vi "SLL DE DO LV2 Global.vi"(6 "DO State Array":bool[](array[boolean]), 7 "DO Option":T2, 8 "Error In":errorcluster, 9 "DO State":bool, 10 "DO Channel Name Array":T1[](array[typedef]), 11 "DO Channel Name":T1) -> (0 "error out":errorcluster, 2 "Digital Array Status":bool[](array[boolean]), 3 "Digital Line Status":bool, 4 "Element Wrote":string)   [LabVIEW 2013]
uses:
  Controls/SLL DE DO Global Options.ctl
  Controls/SLL DE List of Digital Outputs.ctl
  Controls/SLL DE DO Command LV2Global Options.ctl
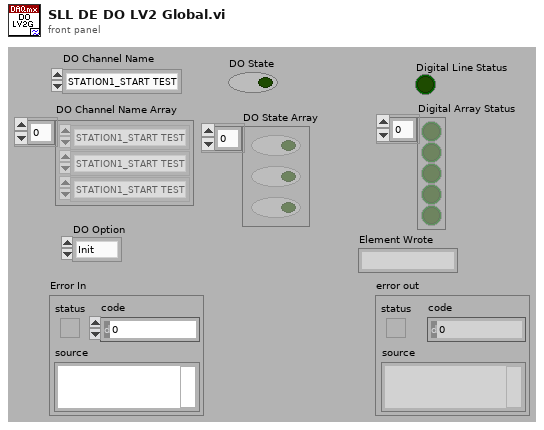
[diagram p1: front panel]
types:
  T1 = typedef "SLL DE List of Digital Outputs.ctl" = enum16{"STATION1_START TEST", "STATION1_STOP TEST", "STATION1_LIGHT1", "STATION1_LIGHT2", "STATION1_LIGHT3", "STATION1_SELECT_TEST", "STATION2_START TEST", "STATION2_STOP TEST", "STATION2_LIGHT1", "STATION2_LIGHT2", "STATION2_LIGHT3", "STATION2_SELECT_TEST", "STATION3_START TEST", "STATION3_STOP TEST", "STATION3_LIGHT1", "STATION3_LIGHT2", "STATION3_LIGHT3", "STATION3_SELECT_TEST", "STATION4_START TEST", "STATION4_STOP TEST", "STATION4_LIGHT1", "STATION4_LIGHT2", "STATION4_LIGHT3", "STATION4_SELECT_TEST"}
  T2 = typedef "SLL DE DO Global Options.ctl" = enum16{"Init", "Write Line", "Write Array", "Write Full Status", "Read Line", "Read Array", "Read Full Status", "Restart DO", "Send to Safe Mode", "Stop DO"}
  T3 = typedef "SLL DE DO Command LV2Global Options.ctl" = enum16{"Init/Register Events", "Get Event Refnum", "Fire Event", "Destroy Event"}
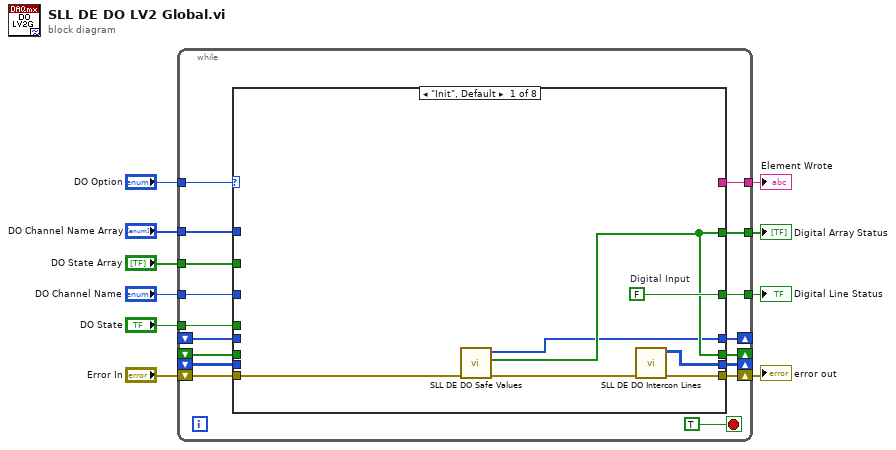
[diagram p0: block diagram]
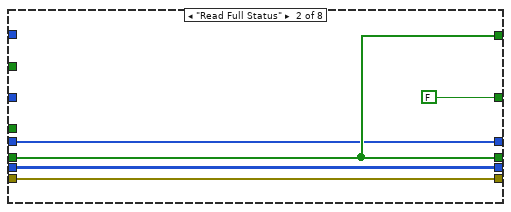
[diagram p2: hidden frame]
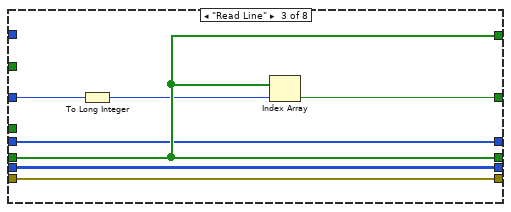
[diagram p3: hidden frame]
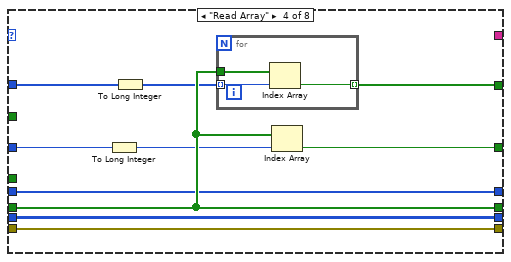
[diagram p4: hidden frame]
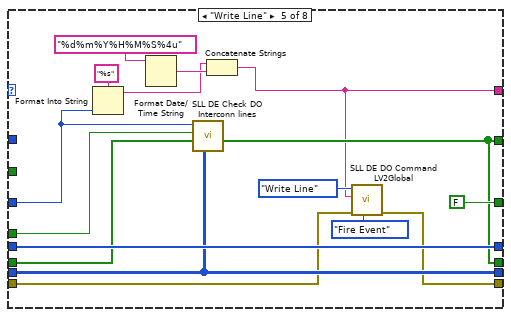
[diagram p5: hidden frame]
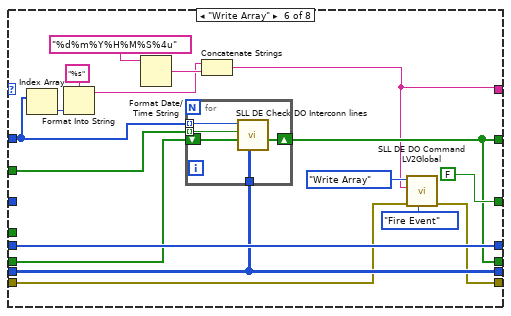
[diagram p6: hidden frame]
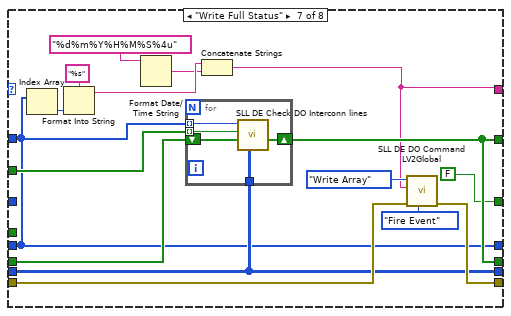
[diagram p7: hidden frame]
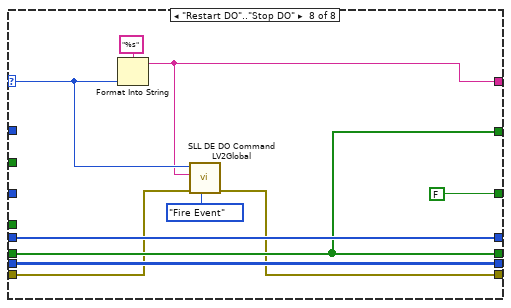
[diagram p8: hidden frame]
diagram:
  n1 = while {
    shift-right: [w26] -> _
    shift-left: _ -> [w25]
    tunnel: "DO Channel Name Array" -> [w24]
    tunnel: "DO Channel Name" -> [w23]
    tunnel: [w22] -> w8
    tunnel: [w21] -> w7
    shift-right: [w19] -> w5
    shift-left: "Error In" -> [w20]
    tunnel: "DO State Array" -> [w18]
    tunnel: "DO State" -> [w17]
    tunnel: "DO Option" -> [w16]
    shift-right: [w15] -> _
    shift-left: _ -> [w14]
    shift-right: [w13] -> _
    shift-left: _ -> [w12]
    tunnel: [w11] -> w1
    stop <- TRUE stop-if-true
    n2 = case shown="\"Init\", Default" w16 {
      selector: w16 -> [_ _ _ _ _ _ _ w122]
      tunnel: [w30 w39 w44 w54 w71 w82 w101 w124] -> w26
      tunnel: w25 -> [_ w39 w44 w54 w70 w81 w105 w124]
      tunnel: w24 -> [_ _ _ w48 _ w84 _ _]
      tunnel: w23 -> [_ _ w46 w53 w63 _ _ _]
      tunnel: [w34 FALSE ("Digital Input") w45 w52 FALSE ("Digital Input") FALSE ("Digital Input") FALSE ("Digital Input") FALSE ("Digital Input")] -> w22
      tunnel: [w30 w39 w44 w56 w71 w82 w101 w124] -> w21
      tunnel: w20 -> [w28 w37 w43 w55 w65 w77 w106 w121]
      tunnel: [w33 w37 w43 w55 w64 w76 w103 w120] -> w19
      tunnel: w18 -> [_ _ _ _ _ w91 w104 _]
      tunnel: w17 -> [_ _ _ _ w73 _ _ _]
      tunnel: [w29 w36 w41 w50 w74 w90 w98 w126] -> w15
      tunnel: w14 -> [_ w36 w41 w50 w74 w90 w98 w126]
      tunnel: [w32 w35 w40 w49 w72 w89 w102 w127] -> w13
      tunnel: w12 -> [_ w35 w40 w49 w72 w89 w102 w127]
      tunnel: [_ _ _ _ w61 w78 w99 w119] -> w11
      frame "Init", Default {
        w34 = FALSE  # Digital Input
        n3 = call "SLL DE DO Safe Values.vi"("error in (no error)"=w28) -> ("error out"=w31:errorcluster, "DO Safe Values"=w30:bool[], "DO Name"=w29:T1[])  [unwired: 8 in]
        n4 = call "SLL DE DO Intercon Lines.vi"("Error In"=w31) -> ("Error Out"=w33:errorcluster, "DO Name"=w32:T1[][])  [unwired: 9 in]
      }
      frame "Read Full Status" {
      }
      frame "Read Line" {
        n5 = To Long Integer(number=w46) -> (32bit integer=w42:i32)
        n6 = Index Array(array=w44, index=w42) -> (element=w45:bool)
      }
      frame "Read Array" {
        n7 = To Long Integer(number=w53) -> (32bit integer=w51:i32)
        n8 = To Long Integer(number=w48) -> (32bit integer=w47:i32[])
        n9 = for {
          tunnel: w54 -> [w59]
          tunnel: w47 -> [w58] mode=indexing
          tunnel: [w57] -> w56 mode=indexing
          n10 = Index Array(array=w59, index=w58) -> (element=w57:bool)
        }
        n11 = Index Array(array=w54, index=w51) -> (element=w52:bool)
      }
      frame "Write Line" {
        n12 = Format Into String(format string="%s", w63) -> (resulting string=w67:string)  [unwired: 2 in, 1 out]
        n13 = Format Date/Time String(time format string (%c)="%d%m%Y%H%M%S%4u") -> (date/time string=w68:string)  [unwired: 2 in]
        n14 = call "SLL DE Check DO Interconn lines.vi"("DO Interconnected lines"=w72, "DO State Array In"=w70, "DO State"=w73, "DO Channel Name"=w63) -> ("DO State Arra Out"=w71:bool[])  [unwired: 7 in]
        n15 = Concatenate Strings(w67, w68) -> (w61:string)
        n16 = call "SLL DE DO Command LV2Global.vi"("Option"=SLL_DE_DO_Command_LV2Global_Options."Fire Event", "Error in (no error)"=w65, "Execute For"=w61, "DO Option"=SLL_DE_DO_Global_Options."Write Line") -> ("Error out"=w64:errorcluster)  [unwired: 6 in, 1 out]
      }
      frame "Write Array" {
        n17 = Index Array(array=w84) -> (element=w83:T1)  [unwired: 1 in]
        n18 = Format Into String(format string="%s", w83) -> (resulting string=w86:string)  [unwired: 2 in, 1 out]
        n19 = Format Date/Time String(time format string (%c)="%d%m%Y%H%M%S%4u") -> (date/time string=w87:string)  [unwired: 2 in]
        n20 = for {
          tunnel: w91 -> [w96] mode=indexing
          shift-right: [w94] -> w82
          shift-left: w81 -> [w97]
          tunnel: w84 -> [w95] mode=indexing
          tunnel: w89 -> [w93]
          n21 = call "SLL DE Check DO Interconn lines.vi"("DO Interconnected lines"=w93, "DO State Array In"=w97, "DO State"=w96, "DO Channel Name"=w95) -> ("DO State Arra Out"=w94:bool[])  [unwired: 7 in]
        }
        n22 = Concatenate Strings(w86, w87) -> (w78:string)
        n23 = call "SLL DE DO Command LV2Global.vi"("Option"=SLL_DE_DO_Command_LV2Global_Options."Fire Event", "Error in (no error)"=w77, "Execute For"=w78, "DO Option"=SLL_DE_DO_Global_Options."Write Array") -> ("Error out"=w76:errorcluster)  [unwired: 6 in, 1 out]
      }
      frame "Write Full Status" {
        n24 = Index Array(array=w98) -> (element=w111:T1)  [unwired: 1 in]
        n25 = Format Into String(format string="%s", w111) -> (resulting string=w109:string)  [unwired: 2 in, 1 out]
        n26 = Format Date/Time String(time format string (%c)="%d%m%Y%H%M%S%4u") -> (date/time string=w108:string)  [unwired: 2 in]
        n27 = for {
          tunnel: w104 -> [w117] mode=indexing
          shift-right: [w115] -> w101
          shift-left: w105 -> [w118]
          tunnel: w98 -> [w116] mode=indexing
          tunnel: w102 -> [w114]
          n28 = call "SLL DE Check DO Interconn lines.vi"("DO Interconnected lines"=w114, "DO State Array In"=w118, "DO State"=w117, "DO Channel Name"=w116) -> ("DO State Arra Out"=w115:bool[])  [unwired: 7 in]
        }
        n29 = Concatenate Strings(w109, w108) -> (w99:string)
        n30 = call "SLL DE DO Command LV2Global.vi"("Option"=SLL_DE_DO_Command_LV2Global_Options."Fire Event", "Error in (no error)"=w106, "Execute For"=w99, "DO Option"=SLL_DE_DO_Global_Options."Write Array") -> ("Error out"=w103:errorcluster)  [unwired: 6 in, 1 out]
      }
      frame "Restart DO".."Stop DO" {
        n31 = Format Into String(format string="%s", w122) -> (resulting string=w119:string)  [unwired: 2 in, 1 out]
        n32 = call "SLL DE DO Command LV2Global.vi"("Option"=SLL_DE_DO_Command_LV2Global_Options."Fire Event", "Error in (no error)"=w121, "Execute For"=w119, "DO Option"=w122) -> ("Error out"=w120:errorcluster)  [unwired: 6 in, 1 out]
      }
    }
  }
  "error out" <- w5
  "Digital Line Status" <- w8
  "Digital Array Status" <- w7
  "Element Wrote" <- w1
